vi "ReadingAttributes.vi"(0 "reference in":refnum<class "MyG#SubClass.lvclass">, 5 "error in (no error)":errorcluster) -> (14 "reference out":refnum<class "MyG#SubClass.lvclass">, 15 "MyAttribute":dbl, 16 "MySubAttribute":dbl, 19 "error out":errorcluster)   [LabVIEW 2020, in "MyG#SubClass.lvclass"]
uses:
  MyG#SubClass.lvclass
  C:/Program Files (x86)/National Instruments/LabVIEW 2020/examples/AddQ/G#/CreateDestroy/MyG#Class_class/MyG#Class.lvclass
  MyG#Class_class/MyG#Class.lvclass
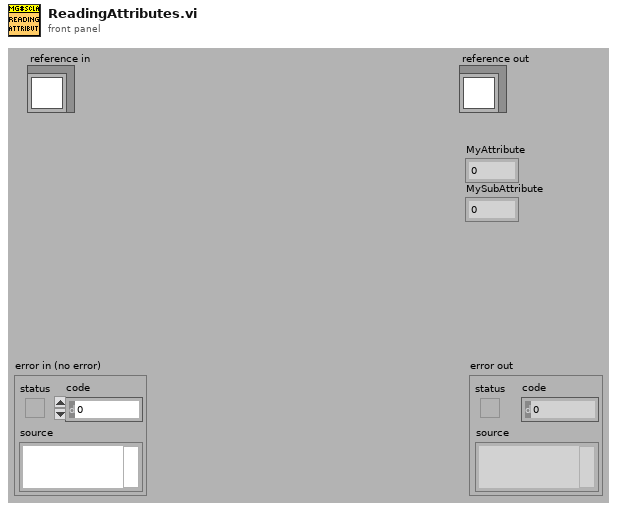
[diagram p1: front panel]
types:
  T1 = typedef "MyG#SubClass.lvclass/ObjectAttributes.ctl" = cluster{"MySubAttribute":dbl}
  T2 = typedef "MyG#Class.lvclass/ObjectAttributes.ctl" = cluster{"MyAttribute":dbl}
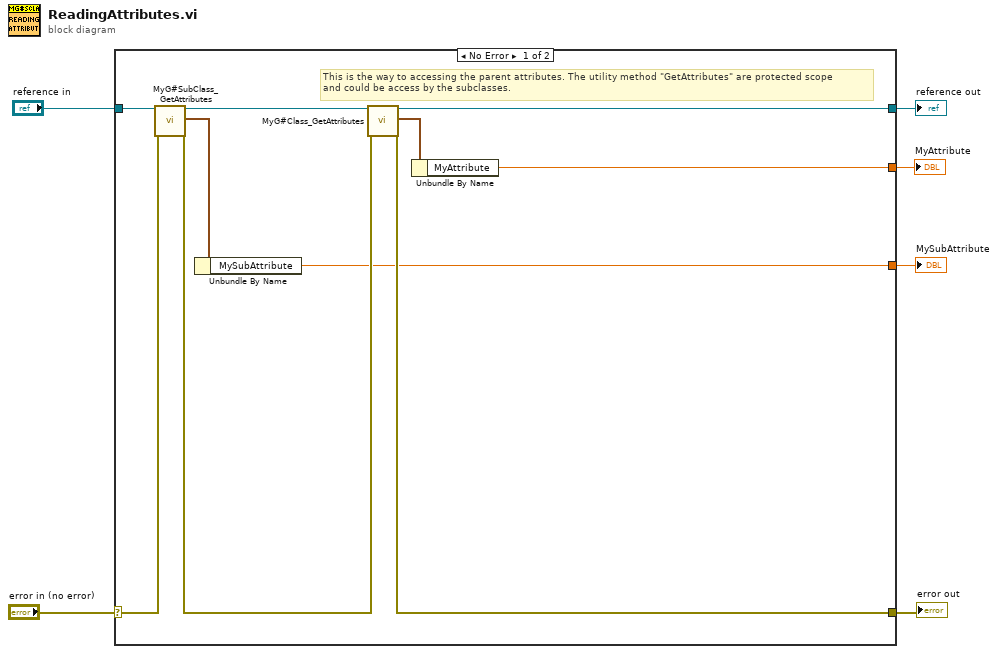
[diagram p0: block diagram]
diagram:
  n1 = case shown="No Error" "error in (no error)" {
    selector: "error in (no error)" -> [w16 w18]
    tunnel: [w10 w18] -> w5
    tunnel: [w12 w17] -> w3
    tunnel: "reference in" -> [w14 w17]
    tunnel: [w8 _] -> w2
    tunnel: [w7 _] -> w1
    frame No Error {
      # "This is the way to accessing the parent attributes. The utility method \"GetAttributes\" are protected scope\nand could be access by the subclasses."
      n2 = call "MyG#SubClass_GetAttributes.vi"("reference in"=w14, "error in (no error)"=w16) -> ("reference out"=w13:refnum<class "MyG#SubClass.lvclass">, "attributes"=w15:T1, "error out"=w11:errorcluster)  [unwired: 14 in, 1 out]
      n3 = Unbundle By Name(w15) -> ("MySubAttribute"=w7:dbl)
      n4 = call "MyG#Class_GetAttributes.vi"("reference in"=w13, "error in (no error)"=w11) -> ("reference out"=w12:refnum<class "MyG#SubClass.lvclass">, "attributes"=w9:T2, "error out"=w10:errorcluster)  [unwired: 14 in, 1 out]
      n5 = Unbundle By Name(w9) -> ("MyAttribute"=w8:dbl)
    }
    frame Error {
    }
  }
  "error out" <- w5
  "reference out" <- w3
  "MyAttribute" <- w2
  "MySubAttribute" <- w1
